vi "DroneCameraSnap.vi"() -> ()   [LabVIEW 2017]
uses:
  <vilib>/LVH/AR Drone Toolkit/Decode NavData/Typedefs/NavData Demo.ctl
  <vilib>/LVH/AR Drone Toolkit/AR Drone.lvlib
panel:
  in  "Snap":bool
  in  "Setup Parameters":T1={"Drone IP address"="192.168.1.1", "Home IP address"="192.168.1.2", "Flight Mode"=enum."INDOOR MODE", "Mounted Hull"=enum."INDOOR HULL", "Video Camera"=2, "Max Altitude (m)"=3.0, "Max Pitch and Roll Angle (deg)"=10.0, "Max Vertical Speed (m/s)"=0.7, "Max Yaw Speed (deg/s)"=100.0} {"Video Camera" items=["Bottom Camera"=1, "Front Camera"=0, "Front in Bottom"=3, "Bottom in Front"=2]}
  out "Video Stream":picture
  out "NavData Out":T2
  out "Battery Remaining":dbl(slide) scale=0.0..100.0
  in  "Hover":bool
  in  "Take Off/Land":bool
  in  "Emergency Landing":bool
  in  "stop 2":bool
  in  "Control Cluster":T3 {"Yaw Speed" scale=-1.0..1.0; "Vertical Speed" scale=-1.0..1.0; "Pitch" scale=-1.0..1.0; "Roll" scale=-1.0..1.0}
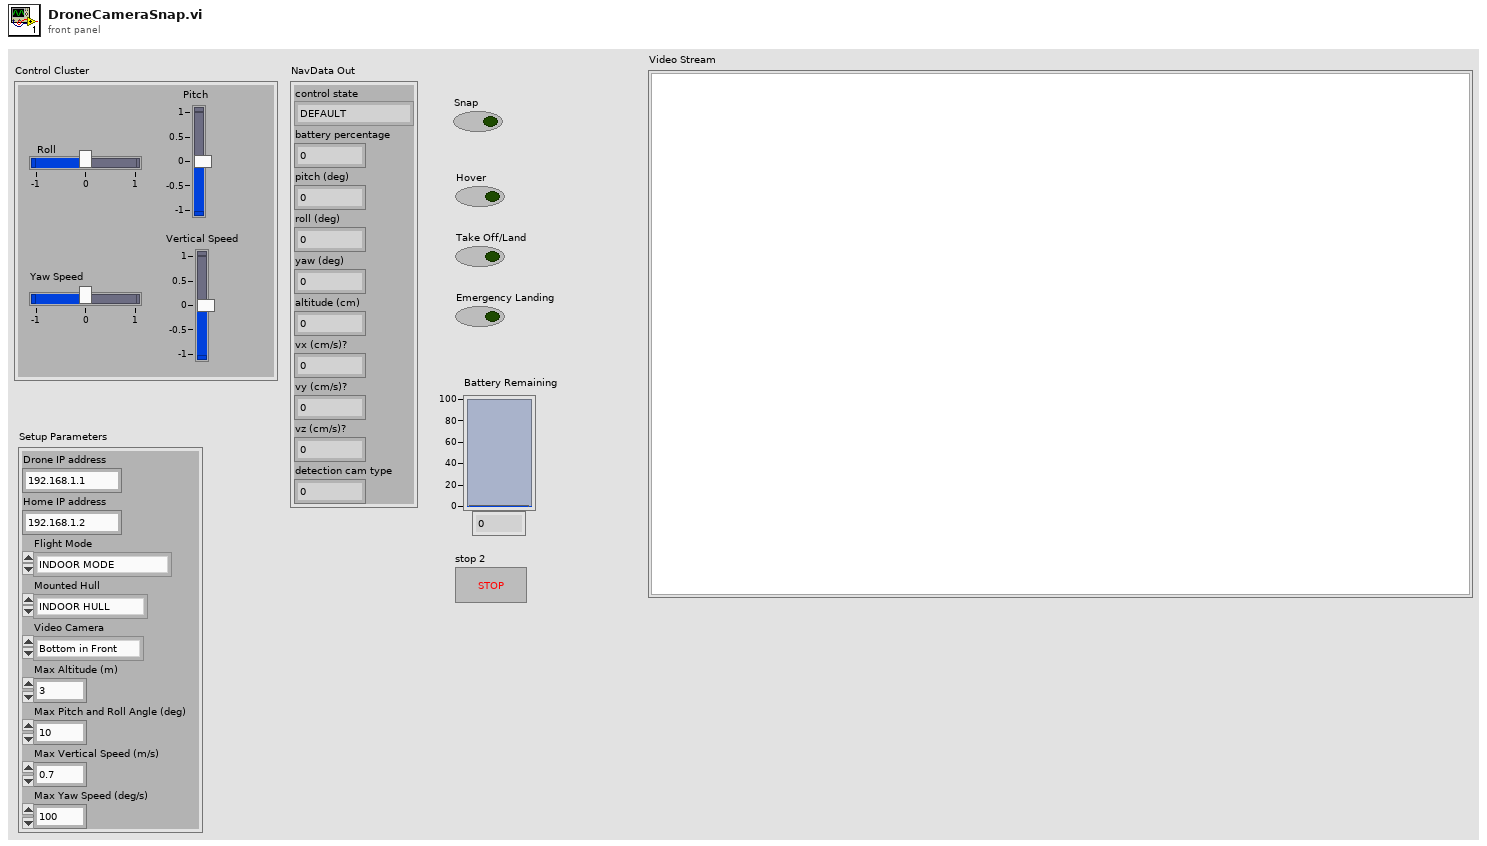
[diagram p1: front panel]
types:
  T1 = cluster{"Drone IP address":string, "Home IP address":string, "Flight Mode":enum8{"OUTDOOR MODE", "INDOOR MODE"}, "Mounted Hull":enum8{"OUTDOOR HULL", "INDOOR HULL"}, "Video Camera":u8, "Max Altitude (m)":sgl, "Max Pitch and Roll Angle (deg)":sgl, "Max Vertical Speed (m/s)":sgl, "Max Yaw Speed (deg/s)":sgl}
  T2 = typedef "AR Drone.lvlib/NavData Demo.ctl" = cluster{"control state":enum32{"DEFAULT", "INIT", "LANDING", "FLYING", "HOVERING", "TEST", "TRANS_TAKEOFF", "TRANS_GOTOFIX", "TRANS_LANDING"}, "battery percentage":u32, "pitch (deg)":sgl, "roll (deg)":sgl, "yaw (deg)":sgl, "altitude (cm)":u32, "vx (cm/s)?":sgl, "vy (cm/s)?":sgl, "vz (cm/s)?":sgl, "detection cam type":u32}
  T3 = cluster{"Roll":sgl, "Pitch":sgl, "Vertical Speed":sgl, "Yaw Speed":sgl}
  T4 = typedef "AR Drone.lvlib/AR Drone Resource.ctl" = cluster{"UDP Control Connection":refnum<k16>, "UDP NavData Connection":refnum<k16>, "UDP Video Connection (Drone 1.0)":refnum<k16>, "TCP Video Connection (Drone 2.0)":refnum<k5>, "TCP Control Port Connection":refnum<k5>, "Drone IP address":string, "Drone Command Port":u16, "Drone NavData Port":u16, "Drone Vid Stream Port":u16, "Drone TCP Control Port":u16, "Home IP address":string, "Home Command Port":u16, "Home NavData Port":u16, "Home Vid Stream Port":u16, "Drone Version":i32, "Drone Index":dbl}
  T5 = typedef "IMAQ Image.ctl" = refnum<image>
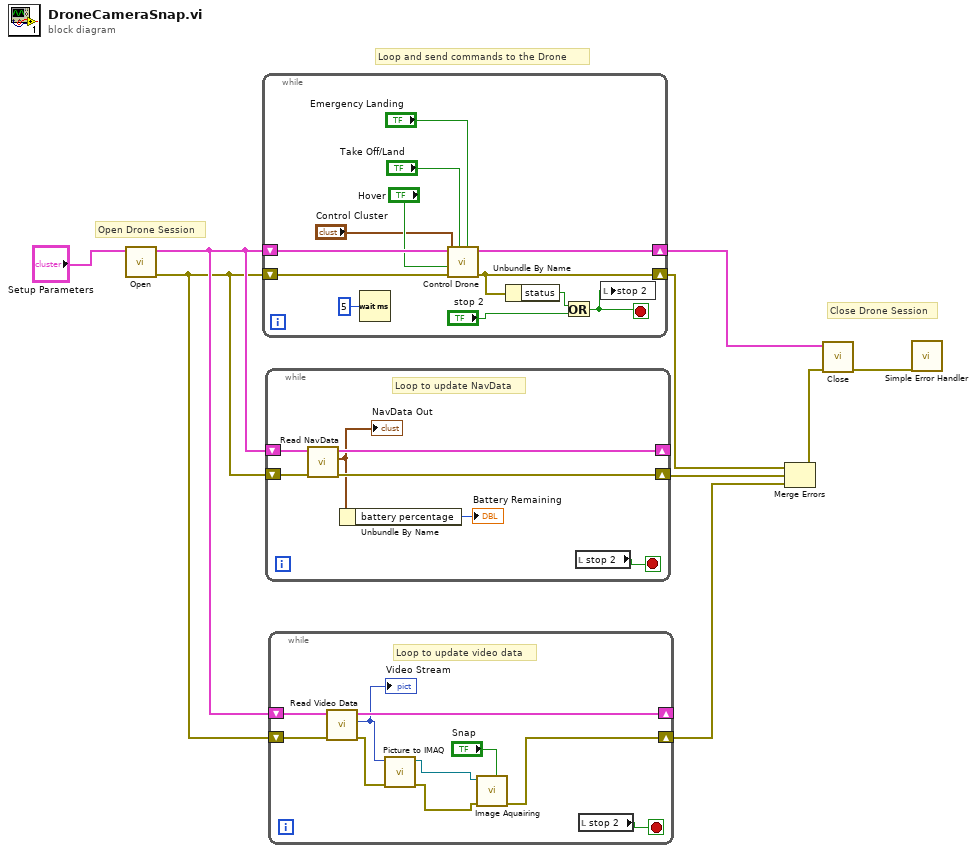
[diagram p0: block diagram]
diagram:
  # "Close Drone Session"
  # "Loop and send commands to the Drone"
  # "Open Drone Session"
  n1 = call <vilib>:"Open.vi"("Setup Parameters"="Setup Parameters") -> ("error out"=w6:errorcluster, "AR Drone Resource"=w7:T4)  [unwired: 9 in]
  n2 = while {
    shift-right: [w16] -> w9
    shift-left: w7 -> [w20]
    shift-right: [w11] -> w2
    shift-left: w6 -> [w21]
    stop <- w10 stop-if-true
    n3 = Wait (ms)(milliseconds to wait=u32 5) -> ()  [unwired: 1 out]
    n4 = call <vilib>:"Control Drone.vi"("Emergency Landing"="Emergency Landing", "Takeoff/Land"="Take Off/Land", "error in (no error)"=w21, "Hover"="Hover", "Control Cluster"="Control Cluster", "AR Drone Resource"=w20) -> ("error out"=w11:errorcluster, "AR Drone Resource Out"=w16:T4)  [unwired: 4 in]
    n5 = Unbundle By Name(w11) -> ("status"=w13:bool)
    n6 = Or(x=w13, y="stop 2") -> (x .or. y?=w10:bool)
    n7 = local write "stop 2"(w10) -> ()
  }
  n8 = while {
    shift-right: [w26] -> _
    shift-left: w7 -> [w27]
    shift-right: [w24] -> w3
    shift-left: w6 -> [w25]
    stop <- w28 stop-if-true
    # "Loop to update NavData"
    n9 = call <vilib>:"Read NavData.vi"("error in (no error)"=w25, "AR Drone Resource"=w27) -> ("error out"=w24:errorcluster, "NavData Out"=w23:T2, "AR Drone Resource Out"=w26:T4)  [unwired: 7 in]
    "NavData Out" <- w23
    n10 = Unbundle By Name(w23) -> ("battery percentage"=→"Battery Remaining":u32)
    n11 = local read "stop 2"() -> (w28:bool)
  }
  n12 = while {
    shift-right: [w35] -> _
    shift-left: w7 -> [w37]
    shift-right: [w30] -> w4
    shift-left: w6 -> [w36]
    stop <- w38 stop-if-true
    # "Loop to update video data"
    n13 = call <vilib>:"Read Video Data.vi"("error in (no error)"=w36, "AR Drone Resource"=w37) -> ("error out"=w34:errorcluster, "Video Stream"=w33:picture, "AR Drone Resource Out"=w35:T4)  [unwired: 7 in]
    "Video Stream" <- w33
    n14 = call "Picture to IMAQ.vi"("Error In"=w34, "picture"=w33) -> ("Error Out"=w31:errorcluster, "Image"=w32:T5)  [unwired: 8 in]
    n15 = call "Image Aquairing.vi"("Boolean"="Snap", "error in (no error)"=w31, "Image In"=w32) -> ("error out"=w30:errorcluster)  [unwired: 8 in]
    n16 = local read "stop 2"() -> (w38:bool)
  }
  n17 = Merge Errors(w2, w3, w4) -> (w5:errorcluster)
  n18 = call <vilib>:"Close.vi"("error in (no error)"=w5, "AR Drone Resource"=w9) -> ("error out"=w8:errorcluster)  [unwired: 9 in]
  n19 = call <vilib>:"Simple Error Handler.vi"("error in (no error)"=w8) -> ()  [unwired: 4 in, 5 out]
